vi "release entry.vi"(8 "error in (no error)":errorcluster, 11 "entry":T1) -> (0 "error out":errorcluster)   [LabVIEW 2024, in "controls manager.lvlib"]
uses:
  controls manager.lvlib
  entry type.ctl
  control.ctl
  controls plan.ctl
  key value pair.ctl
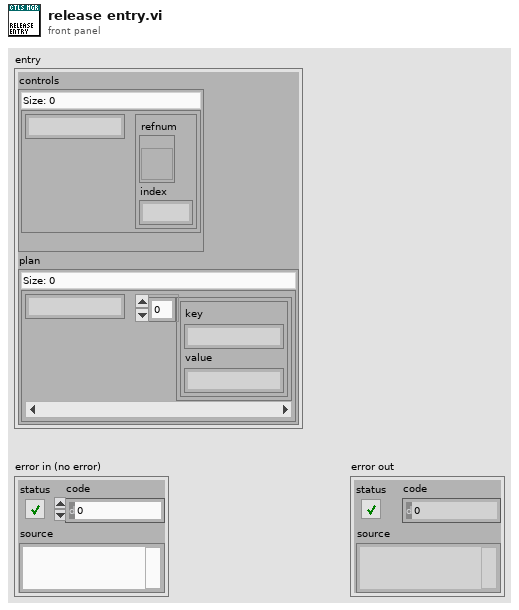
[diagram p1: front panel]
types:
  T1 = typedef "controls manager.lvlib/entry type.ctl" = cluster{"controls":map{string, T2}, "plan":T3}
  T2 = typedef "controls manager.lvlib/control.ctl" = cluster{"refnum":refnum<vi>, "index":i32}
  T3 = typedef "controls manager.lvlib/controls plan.ctl" = map{string, T4[]}
  T4 = typedef "controls manager.lvlib/key value pair.ctl" = cluster{"key":string, "value":string}
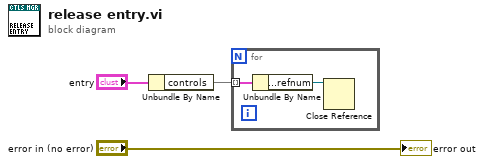
[diagram p0: block diagram]
diagram:
  n1 = Unbundle By Name("entry") -> ("controls"=w1:map{string, T2})
  n2 = for {
    tunnel: w1 -> [w5] mode=indexing
    n3 = Unbundle By Name(w5) -> ("control.refnum"=w4:refnum<vi>)
    n4 = Close Reference(reference=w4) -> ()  [unwired: 1 in, 1 out]
  }
  "error out" <- "error in (no error)"
